vi "create stat file.vi"() -> ()   [LabVIEW 2020]
panel:
  in  "gain":bool
  in  "binning":u16(ring)=2 items=["X 1", "X 2", "X 4", "X 8"]
  in  "exposure [ms]":u32=20
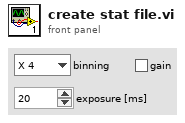
[diagram p1: front panel]
types:
  T1 = enum16{"open", "replace", "create", "open or create", "replace or create", "replace or create with confirmation"}
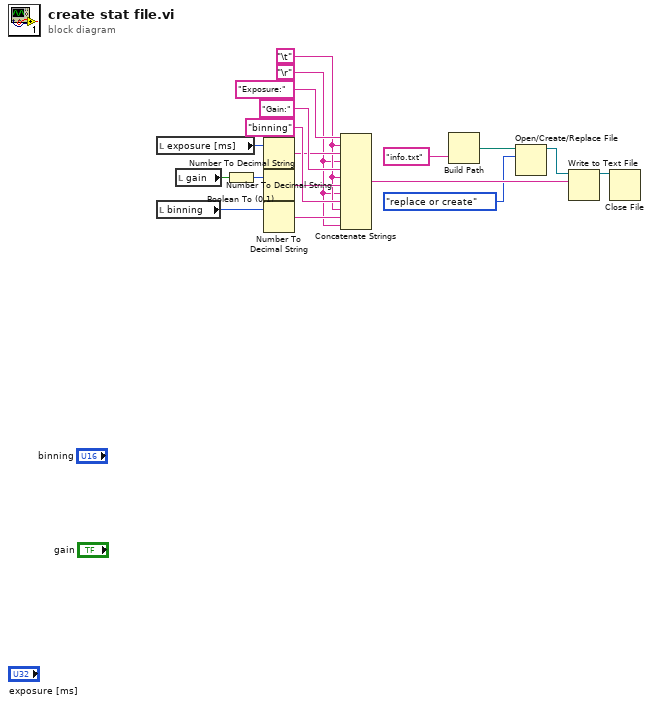
[diagram p0: block diagram]
diagram:
  w1 = "\r"
  w2 = "\t"
  n1 = local read "exposure [ms]"() -> (w9:u32)
  n2 = local read "binning"() -> (w11:u16)
  n3 = local read "gain"() -> (w10:bool)
  n4 = Boolean To (0,1)(Boolean=w10) -> (0, 1=w12:i16)
  n5 = Number To Decimal String(number=w9) -> (decimal integer string=w14:string)  [unwired: 1 in]
  n6 = Number To Decimal String(number=w12) -> (decimal integer string=w16:string)  [unwired: 1 in]
  n7 = Number To Decimal String(number=w11) -> (decimal integer string=w18:string)  [unwired: 1 in]
  n8 = Concatenate Strings("Exposure:", w2, w14, w1, "Gain:", w2, w16, w1, "binning", w2, w18, w1) -> (w8:string)
  n9 = Build Path(name or relative path="info.txt") -> (base path=w19:path, appended path=w4:path)
  n10 = Open/Create/Replace File(file path (use dialog)=w4, operation (0:open)=T1."replace or create") -> (refnum out=w6:refnum<file>)  [unwired: 4 in, 2 out]
  n11 = Write to Text File(file (use dialog)=w6, text=w8) -> (refnum out=w7:refnum<file>)  [unwired: 2 in, 2 out]
  n12 = Close File(refnum=w7) -> ()  [unwired: 1 in, 2 out]
